vi "1 QuadEncoder PositionVelocity.vi"(0 "Encoder Chs":cluster{"ChA":refnum<k21>, "ChB":refnum<k21>}={"ChA"="Chassis1/Mod4/DI4", "ChB"="Chassis1/Mod4/DI5"}, 2 "QuadEncoder Interval (uSec)":u32=1000, 4 "Position Reset":bool) -> (7 "QuadEncoder Packets":u64[](array[numeric]))   [LabVIEW 2010]
uses:
  <vilib>/eio/EIONode/EIONode.xnode
  <vilib>/rvi/eio/nirviEIOImplementation/nirviEIOImplementation.xnode
  <vilib>/rvi/eio/common/nirviEmuClasses.ctl
  <vilib>/rvi/eio/common/nirviEmuTemplateMethod_noerrors.vi
panel:
  out "Velocity (Counts/Interval)":i32
  out "Acceleration (Counts/Interval)":i32
  out "Position (Counts)":i32
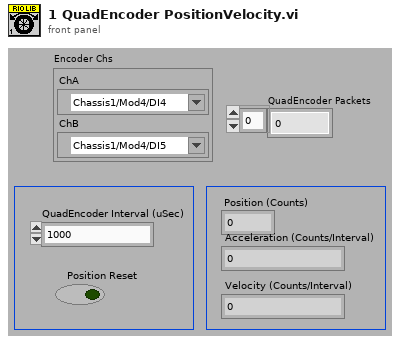
[diagram p1: front panel]
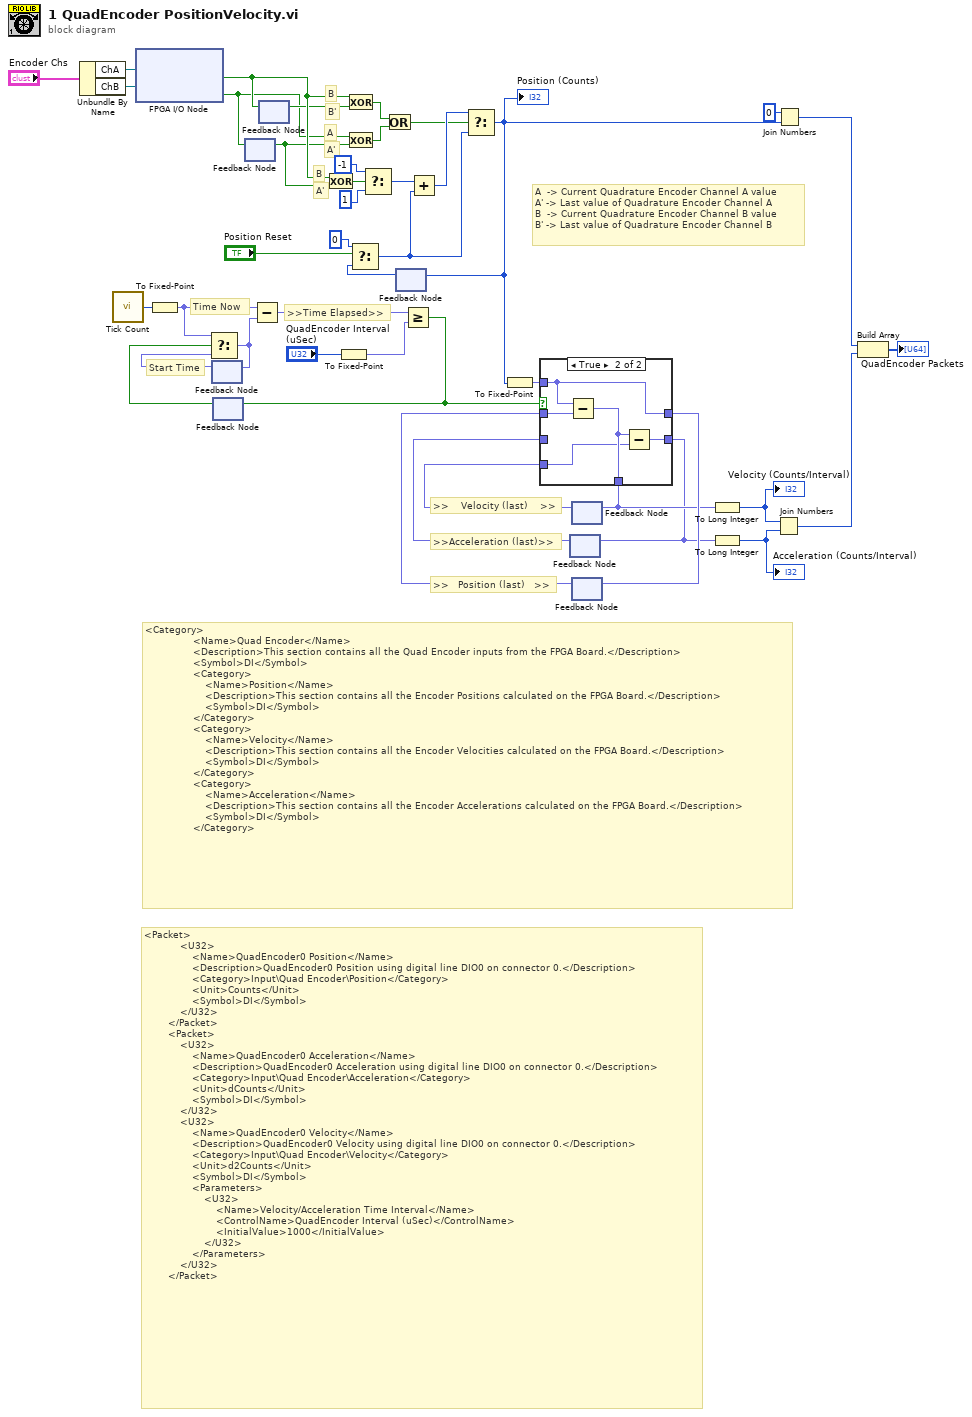
[diagram p0: block diagram]
diagram:
  # "<Category>\n                <Name>Quad Encoder</Name>\n                <Description>This section contains all the Quad Encoder inputs from the FPGA Board.</Description>\n                <Symbol>DI</Symbol>\n                <Category>\n                    <Name>Position</Name>\n                    <Description>This section contains all the Encoder Positions calculated on the FPGA Board.</Description>\n                    <Symbol>DI</Symbol>\n                </Category>\n                <Category>\n                    <Name>Velocity</Name>\n                    <Description>This section contains all the Encoder Velocities calculated on the FPGA Board.</Description>\n                    <Symbol>DI</Symbol>\n                </Category>\n                <Category>\n                    <Name>Acceleration</Name>\n                    <Description>This section contains all the Encoder Accelerations calculated on the FPGA Board.</Description>\n                    <Symbol>DI</Symbol>\n                </Category>"
  # "<Packet>\n            <U32>\n                <Name>QuadEncoder0 Position</Name>\n                <Description>QuadEncoder0 Position using digital line DIO0 on connector 0.</Description>\n                <Category>Input\\Quad Encoder\\Position</Category>\n                <Unit>Counts</Unit>\n                <Symbol>DI</Symbol>\n            </U32>\n        </Packet>\n        <Packet>\n            <U32>\n                <Name>QuadEncoder0 Acceleration</Name>\n                <Description>QuadEncoder0 Acceleration using digital line DIO0 on connector 0.</Description>\n                <Category>Input\\Quad Encoder\\Acceleration</Category>\n                <Unit>dCounts</Unit>\n                <Symbol>DI</Symbol>\n            </U32>\n            <U32>\n                <Name>QuadEncoder0 Velocity</Name>\n                <Description>QuadEncoder0 Velocity using digital line DIO0 on connector 0.</Description>\n                <Category>Input\\Quad Encoder\\Velocity</Category>\n                <Unit>d2Counts</Unit>\n                <Symbol>DI</Symbol>\n                <Parameters>\n                    <U32>\n                        <Name>Velocity/Acceleration Time Interval</Name>\n                        <ControlName>QuadEncoder Interval (uSec)</ControlName>\n                        <InitialValue>1000</InitialValue>\n                    </U32>\n                </Parameters>\n            </U32>\n        </Packet>"
  # "A  -> Current Quadrature Encoder Channel A value\nA' -> Last value of Quadrature Encoder Channel A\nB  -> Current Quadrature Encoder Channel B value\nB' -> Last value of Quadrature Encoder Channel B"
  # ">>Acceleration (last)>>"
  # "Start Time"
  # "A'"
  # "B"
  # "A'"
  # "A"
  # "B'"
  # "B"
  # ">>    Velocity (last)    >>"
  # ">>   Position (last)   >>"
  # "Time Now"
  # ">>Time Elapsed>>"
  n1 = Unbundle By Name("Encoder Chs") -> ("ChA"=w16:refnum<k21>, "ChB"=w15:refnum<k21>)
  n2 = call "Tick Count"() -> ("Tick Count(uSec)"=w18:u32)
  n3 = xnode "FPGA I/O Node"("FPGA I/O In"=w16, "FPGA I/O In"=w15) -> ("I/O Item"=w22:bool, "I/O Item"=w20:bool)  [unwired: 2 out]
  n4 = To Fixed-Point(number=w18) -> (fixed-point=w7:fxp<+,32,32>)  [unwired: 1 in]
  n5 = feedback #1() -> (w28:fxp<+,32,32>)  [unwired: 1 in]
  n6 = feedback #2() -> (w30:bool)  [unwired: 1 in]
  n7 = Select(t=w7, s=w30, f=w28) -> (s? t:f=w5:fxp<+,32,32>)
  n8 = feedback-in #1(w5) -> ()
  n9 = feedback-in #3(w20) -> ()
  n10 = feedback #3() -> (w19:bool)  [unwired: 1 in]
  n11 = Subtract(x=w7, y=w5) -> (x-y=w6:fxp<+,32,32>)
  n12 = feedback-in #4(w22) -> ()
  n13 = feedback #4() -> (w21:bool)  [unwired: 1 in]
  n14 = Exclusive Or(1:w19, 2:w22) -> (0:w33:bool)
  n15 = To Fixed-Point(number="QuadEncoder Interval (uSec)") -> (fixed-point=w4:fxp<+,32,32>)  [unwired: 1 in]
  n16 = Exclusive Or(1:w21, 2:w22) -> (0:w34:bool)
  n17 = Exclusive Or(1:w19, 2:w20) -> (0:w35:bool)
  n18 = Select(t=-1 ("32 bit"), s=w33, f=1 ("32 bit")) -> (s? t:f=w38:i32)
  n19 = Or(x=w34, y=w35) -> (x .or. y?=w32:bool)
  n20 = feedback #5() -> (w31:i32)  [unwired: 1 in]
  n21 = Select(t=0 ("32 bit"), s="Position Reset", f=w31) -> (s? t:f=w40:i32)
  n22 = Greater Or Equal?(x=w6, y=w4) -> (x >= y?=w27:bool)
  n23 = feedback-in #2(w27) -> ()
  n24 = Add(x=w38, y=w40) -> (x+y=w42:i32)
  n25 = Select(t=w42, s=w32, f=w40) -> (s? t:f=w14:i32)
  "Position (Counts)" <- w14
  n26 = feedback-in #5(w14) -> ()
  n27 = To Fixed-Point(number=w14) -> (fixed-point=w3:fxp<+/-,32,32>)  [unwired: 1 in]
  n28 = feedback #6() -> (w24:fxp<+/-,32,32>)  [unwired: 1 in]
  n29 = feedback #7() -> (w25:fxp<+/-,32,32>)  [unwired: 1 in]
  n30 = feedback #8() -> (w26:fxp<+/-,32,32>)  [unwired: 1 in]
  n31 = case shown="True" w27 {
    tunnel: w3 -> [_ w50]
    tunnel: w26 -> [w43 w49]
    tunnel: [w45 w48] -> w12
    tunnel: w25 -> [w45 w47]
    tunnel: [w44 w46] -> w11
    tunnel: w24 -> [w44 _]
    tunnel: [w43 w50] -> w23
    frame False {
    }
    frame True {
      n32 = Subtract(x=w50, y=w49) -> (x-y=w48:fxp<+/-,32,32>)
      n33 = Subtract(x=w48, y=w47) -> (x-y=w46:fxp<+/-,32,32>)
    }
  }
  n34 = feedback-in #6(w11) -> ()
  n35 = feedback-in #7(w12) -> ()
  n36 = feedback-in #8(w23) -> ()
  n37 = To Long Integer(number=w12) -> (32bit integer=w2:i32)
  "Velocity (Counts/Interval)" <- w2
  n38 = To Long Integer(number=w11) -> (32bit integer=w1:i32)
  "Acceleration (Counts/Interval)" <- w1
  n39 = Join Numbers(hi=w2, lo=w1) -> ((hi.lo)=w9:u64)
  n40 = Join Numbers(hi=0, lo=w14) -> ((hi.lo)=w10:u64)
  n41 = Build Array(w10, w9) -> (→"QuadEncoder Packets":u64[])
